vi "1553 Channels to Channel Handles.vi"(8 "error in":errorcluster, 10 "1553 channels":T5[](array[typedef]), 11 "Ballard MIL-STD 1553 custom device in":T2 format="%.0x") -> (0 "error out":errorcluster, 1 "Tx Channels":T2[](array[typedef]) format="%.0x", 2 "Rx Channels":T2[](array[typedef]) format="%.0x", 3 "Ballard MIL-STD 1553 custom device out":T2 format="%.0x", 4 "TX Messages":T1[](array[typedef]) {"Message Section Handle" format="%.0x"; "Parameter Channel Handles" format="%.0x"}, 6 "RX Messages":T1[](array[typedef]) {"Message Section Handle" format="%.0x"; "Parameter Channel Handles" format="%.0x"})   [LabVIEW 2020, in "AIM MIL-STD-1553 Engine.lvlib" / "Implementation.lvlib" / "Execution Unit.lvclass"]
uses:
  Execution Unit.lvclass
  <vilib>/NI VeriStand/Custom Device API/Custom Device Item Ref.ctl
  <vilib>/NI VeriStand/Custom Device API/Custom Device API.lvlib
  1553 Channel Handles.ctl
  Scripting/AIM MIL-STD-1553 Scripting.lvlib
  Parameter Handles.ctl
  Message Handles.ctl
  Shared/Error Count Channel Refs.ctl
  Shared/Direction.ctl
  Custom Device/Compiled Message.ctl
  Custom Device/Custom Device.lvlib
  Shared/Parameter Definition.ctl
  Shared/Address.ctl
  Shared/Terminal Endpoint.ctl
  Shared/Message Type.ctl
  Shared/Message Definition.ctl
  Shared/1553 Channel.ctl
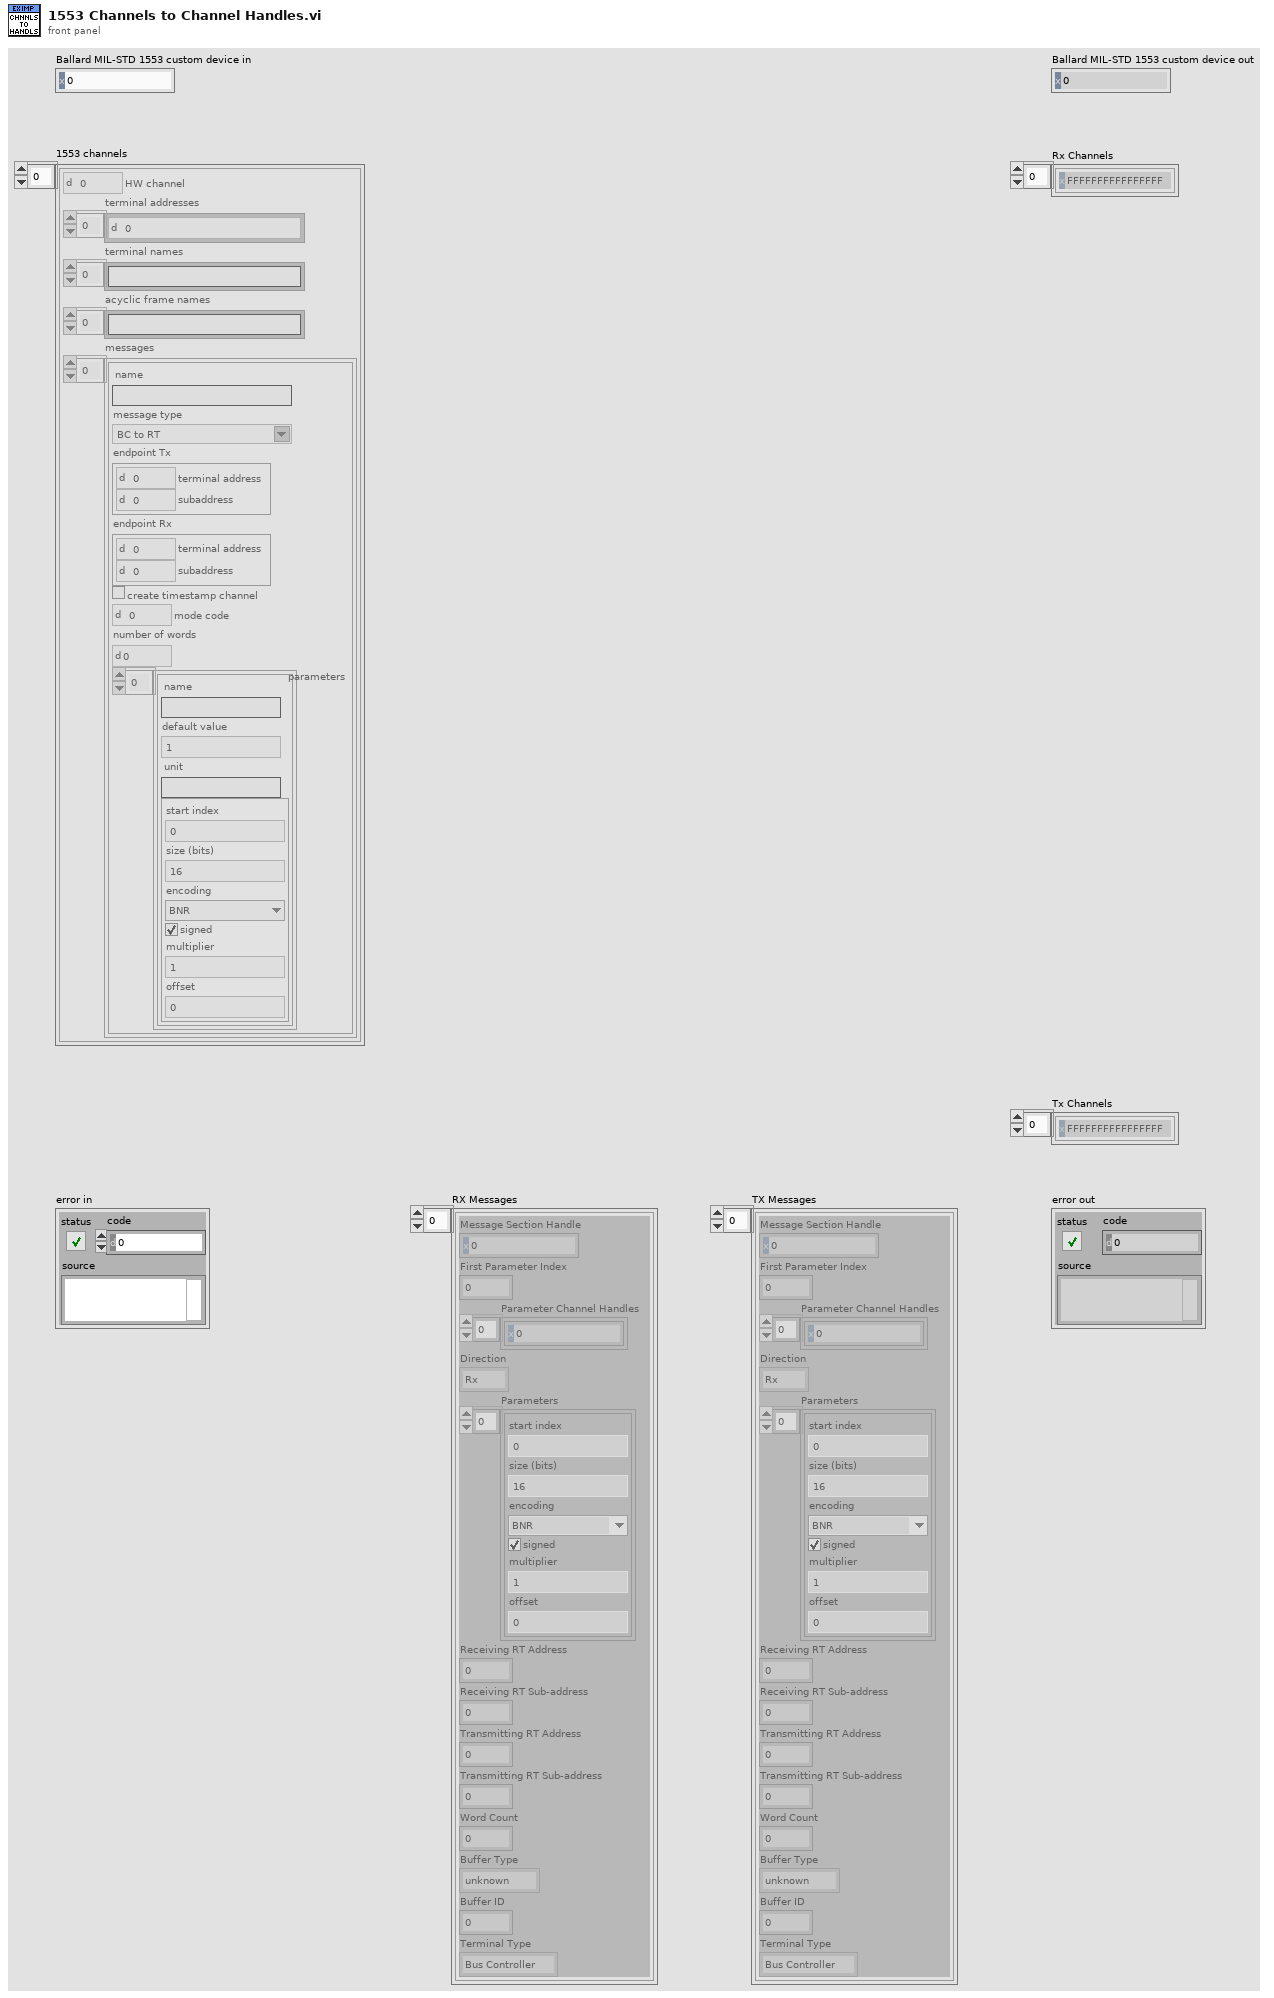
[diagram p1: front panel]
types:
  T1 = typedef "AIM MIL-STD-1553 Engine.lvlib/Custom Device.lvlib/Compiled Message.ctl" = cluster{"Message Section Handle":T2, "First Parameter Index":i32, "Parameter Channel Handles":T2[], "Direction":T3, "Parameters":T4[], "Receiving RT Address":u8, "Receiving RT Sub-address":u8, "Transmitting RT Address":u8, "Transmitting RT Sub-address":u8, "Word Count":u8, "Buffer Type":enum16{"unknown", "BC Message Buffer", "RT Message Buffer"}, "Buffer ID":u16, "Terminal Type":enum16{"Bus Controller", "Remote Terminal"}}
  T2 = typedef "Custom Device API.lvlib/Custom Device Item Ref.ctl" = u64
  T3 = typedef "Direction.ctl" = enum16{"Rx", "Tx"}
  T4 = typedef "Parameter Definition.ctl" = cluster{"start index":i32, "size (bits)":i32, "encoding":enum16{"BNR", "BCD", "Discrete"}, "signed":bool, "multiplier":dbl, "offset":dbl}
  T5 = typedef "1553 Channel.ctl" = cluster{"HW channel":u16, "terminal addresses":T6[], "terminal names":string[], "acyclic frame names":string[], "messages":T7[]}
  T6 = typedef "Address.ctl" = u16
  T7 = typedef "Message Definition.ctl" = cluster{"name":string, "message type":T8, "endpoint Tx":T9, "endpoint Rx":T9, "create timestamp channel":bool, "mode code":u16, "number of words":u16, "parameters":cluster{"name":string, "default value":dbl, "unit":string, "parameter definition":T4}[]}
  T8 = typedef "Message Type.ctl" = string
  T9 = typedef "Terminal Endpoint.ctl" = cluster{"terminal address":T6, "subaddress":T6}
  T10 = typedef "AIM MIL-STD-1553 Engine.lvlib/Implementation.lvlib/Execution Unit.lvclass/1553 Channel Handles.ctl" = cluster{"messages":T11[], "error count channel refs":T13, "terminal status channels":T2[]}
  T11 = typedef "AIM MIL-STD-1553 Engine.lvlib/Implementation.lvlib/Execution Unit.lvclass/Message Handles.ctl" = cluster{"parameters":T12[], "timestamps":T2[], "Tx status handles":T2[], "Rx status handles":T2[]}
  T12 = typedef "AIM MIL-STD-1553 Engine.lvlib/Implementation.lvlib/Execution Unit.lvclass/Parameter Handles.ctl" = cluster{"Tx channel handle":T2, "RxRT channel handle":T2, "RxBC channel handle":T2}
  T13 = typedef "Error Count Channel Refs.ctl" = cluster{"general protocol":T2, "improper number of words":T2, "Manchester":T2, "monitor":T2, "parity":T2, "unconfigured frames":T2, "word":T2, "wrong sync":T2}
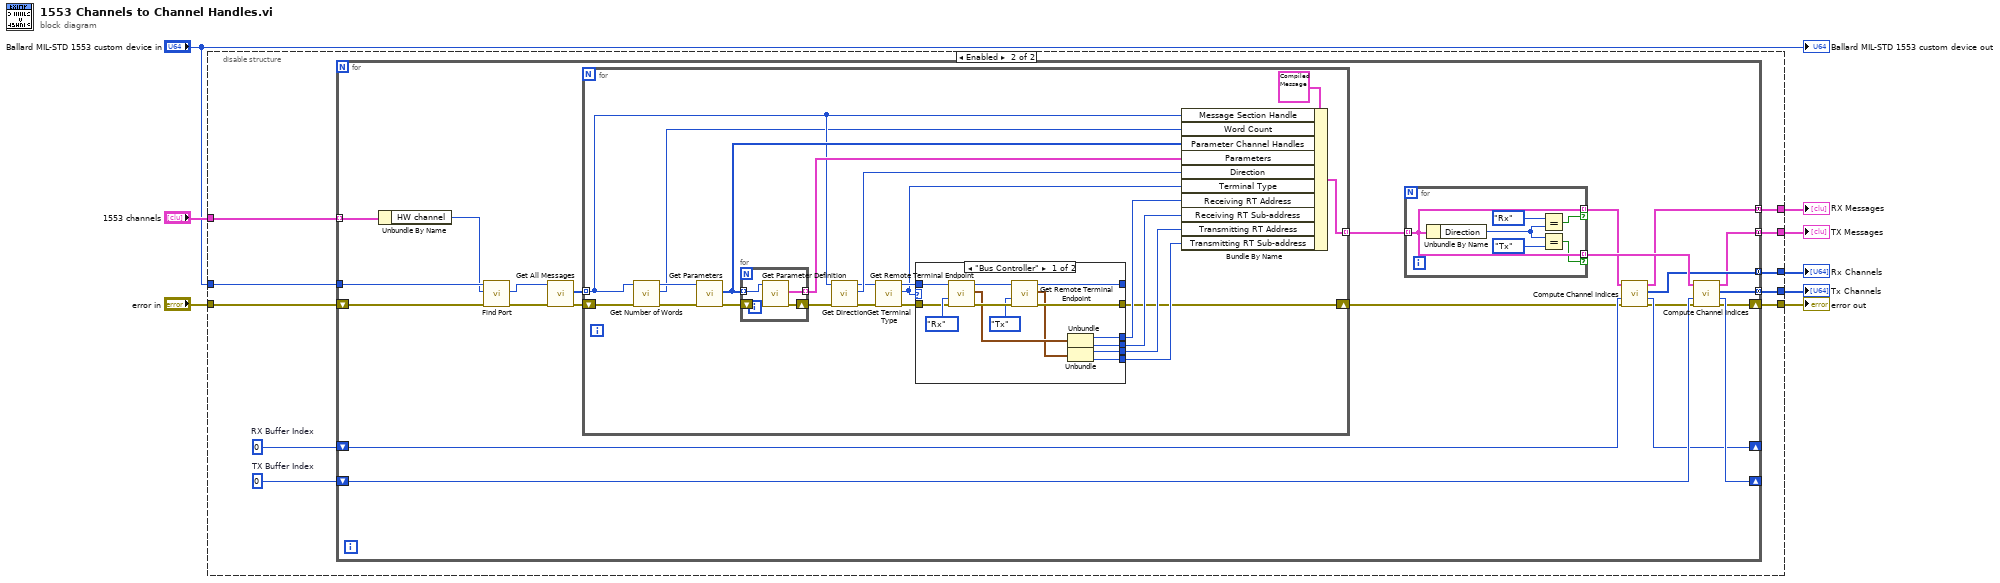
[diagram p0: block diagram]
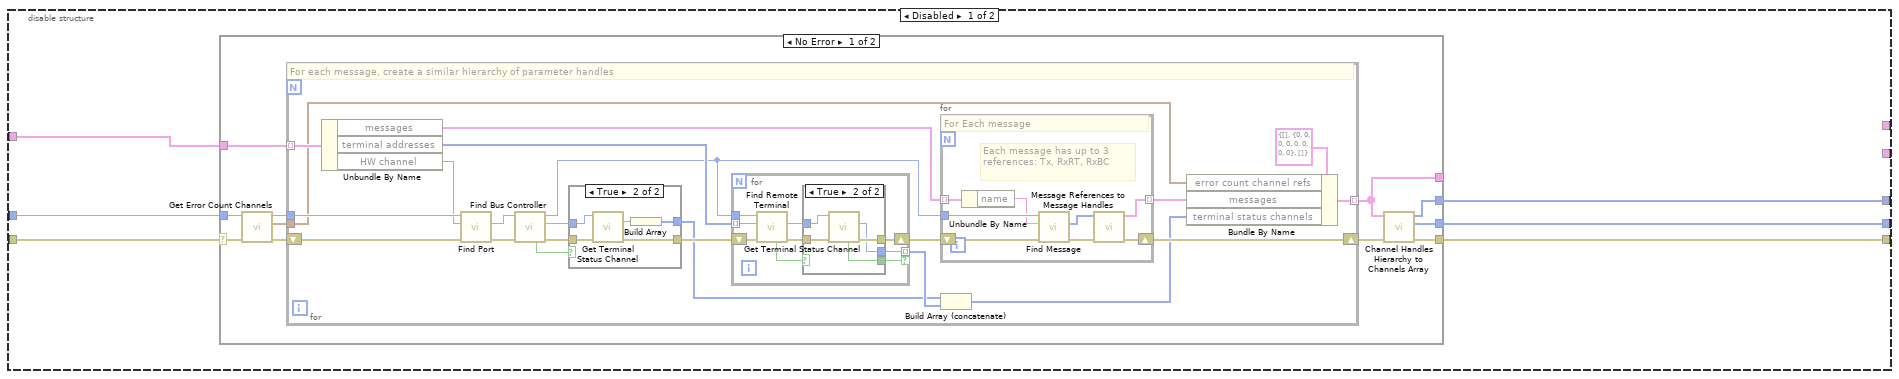
[diagram p2: hidden frame]
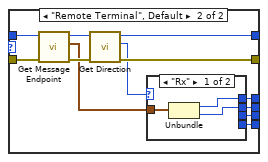
[diagram p6: hidden frame]
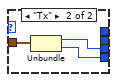
[diagram p7: hidden frame]
diagram:
  n1 = disable-structure shown="Enabled" {
    disable-tunnel: "error in" -> [w14 w89]
    disable-tunnel: "1553 channels" -> [w13 w87]
    disable-tunnel: [w12 w88] -> w6
    disable-tunnel: [w11 w85] -> w5
    disable-tunnel: [w10 w82] -> w4
    disable-tunnel: "Ballard MIL-STD 1553 custom device in" -> [w9 w86]
    disable-tunnel: [_ w81] -> w2
    disable-tunnel: [_ w80] -> w1
    frame Disabled {
      n2 = case shown="No Error" w14 {
        selector: w14 -> [w18 w79]
        tunnel: w13 -> [w25 _]
        tunnel: [w23 w79] -> w12
        tunnel: [w22 _] -> w11
        tunnel: [w21 _] -> w10
        tunnel: [w20 _] -> _
        tunnel: w9 -> [w17 _]
        frame No Error {
          n3 = call "Get Error Count Channels.vi"("error in"=w18, "Ballard MIL-STD-1553 custom device in"=w17) -> ("error out"=w19:errorcluster, "error count channel refs"=w15:T13, "Ballard MIL-STD-1553 custom device out"=w16:T2)  [unwired: 6 in, 1 out]
          n4 = for {
            tunnel: w25 -> [w42] mode=indexing
            shift-right: [w43] -> w24
            shift-left: w19 -> [w40]
            tunnel: [w44] -> w20 mode=indexing
            tunnel: w16 -> [w41]
            tunnel: w15 -> [w26]
            # "For each message, create a similar hierarchy of parameter handles"
            n5 = Unbundle By Name(w42) -> ("messages"=w47:T7[], "terminal addresses"=w38:T6[], "HW channel"=w27:u16)
            n6 = call "Find Port.vi"("error in"=w40, "port number"=w27, "Ballard MIL-STD 1553 custom device in"=w41) -> ("error out"=w36:errorcluster, "port"=w35:T2)  [unwired: 5 in, 2 out]
            n7 = call "Find Bus Controller.vi"("error in"=w36, "port in"=w35) -> ("error out"=w30:errorcluster, "bus controller"=w32:T2, "port out"=w33:T2, "found?"=w31:bool)  [unwired: 6 in]
            n8 = case shown="True" w31 {
              tunnel: w32 -> [_ w53]
              tunnel: w30 -> [w48 w51]
              tunnel: [w48 w50] -> w29
              tunnel: [_ w49] -> w28
              frame False {
              }
              frame True {
                n9 = call "Get Terminal Status Channel.vi"("error in"=w51, "terminal in"=w53) -> ("error out"=w50:errorcluster, "status channel"=w52:T2)  [unwired: 6 in, 2 out]
                n10 = Build Array(w52) -> (w49:T2[])
              }
            }
            n11 = for {
              shift-right: [w59] -> w39
              shift-left: w29 -> [w61]
              tunnel: w33 -> [w62]
              tunnel: w38 -> [w60] mode=indexing
              tunnel: [w55] -> w37 mode=indexing if=w54
              n12 = call "Find Remote Terminal.vi"("error in"=w61, "terminal address"=w60, "port in"=w62) -> ("error out"=w56:errorcluster, "remote terminal"=w57:T2, "found?"=w58:bool)  [unwired: 5 in, 1 out]
              n13 = case shown="True" w58 {
                selector: w58 -> [w63 _]
                tunnel: w57 -> [w64 w70]
                tunnel: w56 -> [w65 w69]
                tunnel: [w65 w68] -> w59
                tunnel: [w64 w67] -> w55
                tunnel: [w63 w66] -> w54
                frame False {
                }
                frame True {
                  n14 = call "Get Terminal Status Channel.vi"("error in"=w69, "terminal in"=w70) -> ("error out"=w68:errorcluster, "status channel"=w67:T2, "found?"=w66:bool)  [unwired: 6 in, 1 out]
                }
              }
            }
            n15 = for {
              tunnel: w47 -> [w77] mode=indexing
              shift-right: [w72] -> w43
              shift-left: w39 -> [w78]
              tunnel: w33 -> [w76]
              tunnel: [w71] -> w45 mode=indexing
              # "Each message has up to 3 references: Tx, RxRT, RxBC"
              # "For Each message"
              n16 = Unbundle By Name(w77) -> ("name"=w75:string)
              n17 = call "Find Message.vi"("error in"=w78, "message name"=w75, "port in"=w76) -> ("error out"=w74:errorcluster, "message refs"=w73:T2[])  [unwired: 5 in, 2 out]
              n18 = call "Message References to Message Handles.vi"("error in"=w74, "message refs"=w73) -> ("error out"=w72:errorcluster, "message handles"=w71:T11)  [unwired: 8 in]
            }
            n19 = Build Array (concatenate)(w28, w37) -> (w34:T2[])
            n20 = Bundle By Name(cluster=T10 {"messages"=[], "error count channel refs"={"general protocol"=0, "improper number of words"=0, "Manchester"=0, "monitor"=0, "parity"=0, "unconfigured frames"=0, "word"=0, "wrong sync"=0}, "terminal status channels"=[]} ("1553 channel handles"), "error count channel refs"=w26, "messages"=w45, "terminal status channels"=w34) -> (w44:T10)
          }
          n21 = call "Channel Handles Hierarchy to Channels Array.vi"("error in"=w24, "1553 channel handles"=w20) -> ("error out"=w23:errorcluster, "Tx Channels"=w22:T2[], "Rx Channels"=w21:T2[])  [unwired: 7 in]
        }
        frame Error {
        }
      }
    }
    frame Enabled {
      w83 = 0  # RX Buffer Index
      w84 = 0  # TX Buffer Index
      n22 = for {
        shift-right: [w92] -> w88
        shift-left: w89 -> [w110]
        tunnel: w87 -> [w111] mode=indexing
        tunnel: w86 -> [w109]
        tunnel: [w100] -> w85 mode=concatenating
        shift-right: [w96] -> _
        shift-left: w83 -> [w97]
        shift-right: [w98] -> _
        shift-left: w84 -> [w99]
        tunnel: [w95] -> w82 mode=concatenating
        tunnel: [w91] -> w81 mode=concatenating
        tunnel: [w90] -> w80 mode=concatenating
        n23 = Unbundle By Name(w111) -> ("HW channel"=w108:u16)
        n24 = call "Find Port.vi"("error in"=w110, "port number"=w108, "Ballard MIL-STD 1553 custom device in"=w109) -> ("error out"=w107:errorcluster, "port"=w106:T2)  [unwired: 5 in, 2 out]
        n25 = call "Get All Messages.vi"("error in"=w107, "port in"=w106) -> ("error out"=w105:errorcluster, "messages"=w104:T2[])  [unwired: 7 in, 1 out]
        n26 = for {
          shift-right: [w124] -> w94
          shift-left: w105 -> [w122]
          tunnel: w104 -> [w123] mode=indexing
          tunnel: [w139] -> w103 mode=indexing
          n27 = call "Get Number of Words.vi"("error in"=w122, "message in"=w123) -> ("error out"=w121:errorcluster, "number of words"=w119:u16, "message out"=w120:T2)  [unwired: 7 in]
          n28 = call "Get Parameters.vi"("error in"=w121, "message in"=w120) -> ("error out"=w136:errorcluster, "parameters"=w135:T2[])  [unwired: 7 in, 1 out]
          n29 = for {
            shift-right: [w175] -> w133
            shift-left: w136 -> [w174]
            tunnel: w135 -> [w173] mode=indexing
            tunnel: [w172] -> w134 mode=indexing
            n30 = call "Get Parameter Definition.vi"("error in"=w174, "parameter in"=w173) -> ("error out"=w175:errorcluster, "parameter definition"=w172:T4)  [unwired: 7 in, 1 out]
          }
          n31 = call "Get Direction.vi"("error in"=w133, "message in"=w123) -> ("error out"=w130:errorcluster, "direction"=w137:T3, "message out"=w129:T2)  [unwired: 6 in, 1 out]
          n32 = call "Get Terminal Type.vi"("error in"=w130, "message in"=w129) -> ("error out"=w132:errorcluster, "terminal type"=w118:enum16{"Bus Controller", "Remote Terminal"}, "message out"=w131:T2)  [unwired: 7 in]
          n33 = case shown="\"Bus Controller\"" w118 {
            tunnel: [w147 w163] -> _
            tunnel: [w146 w162] -> w124
            tunnel: w131 -> [w153 w159]
            tunnel: w132 -> [w151 w158]
            tunnel: [w140 w157] -> w125
            tunnel: [w141 w156] -> w126
            tunnel: [w144 w155] -> w127
            tunnel: [w145 w154] -> w128
            frame "Bus Controller" {
              n34 = call "Get Remote Terminal Endpoint.vi"("error in"=w151, "direction"=Direction."Rx", "message in"=w153) -> ("error out"=w150:errorcluster, "remote terminal"=w143:T9, "message out"=w148:T2)  [unwired: 5 in, 1 out]
              n35 = call "Get Remote Terminal Endpoint.vi"("error in"=w150, "direction"=Direction."Tx", "message in"=w148) -> ("error out"=w146:errorcluster, "remote terminal"=w142:T9, "message out"=w147:T2)  [unwired: 5 in, 1 out]
              n36 = Unbundle(w143) -> ("terminal address"=w145:T6, "subaddress"=w144:T6)
              n37 = Unbundle(w142) -> ("terminal address"=w141:T6, "subaddress"=w140:T6)
            }
            frame "Remote Terminal", Default {
              n38 = call "Get Message Endpoint.vi"("error in"=w158, "message in"=w159) -> ("error out"=w164:errorcluster, "message endpoint"=w160:T9, "message out"=w165:T2)  [unwired: 7 in]
              n39 = call "Get Direction.vi"("error in"=w164, "message in"=w165) -> ("error out"=w162:errorcluster, "direction"=w161:T3, "message out"=w163:T2)  [unwired: 6 in, 1 out]
              n40 = case shown="\"Rx\"" w161 {
                tunnel: w160 -> [w168 w171]
                tunnel: [w167 _] -> w154
                tunnel: [w166 _] -> w155
                tunnel: [_ w170] -> w156
                tunnel: [_ w169] -> w157
                frame "Rx" {
                  n41 = Unbundle(w168) -> ("terminal address"=w167:T6, "subaddress"=w166:T6)
                }
                frame "Tx" {
                  n42 = Unbundle(w171) -> ("terminal address"=w170:T6, "subaddress"=w169:T6)
                }
              }
            }
          }
          n43 = Bundle By Name(cluster=T1 {"Message Section Handle"=18446744073709551615, "First Parameter Index"=0, "Parameter Channel Handles"=[], "Direction"=enum."Rx", "Parameters"=[], "Receiving RT Address"=0, "Receiving RT Sub-address"=0, "Transmitting RT Address"=0, "Transmitting RT Sub-address"=0, "Word Count"=0, "Buffer Type"=enum."unknown", "Buffer ID"=0, "Terminal Type"=enum."Bus Controller"}, "Message Section Handle"=w123, "Word Count"=w119, "Parameter Channel Handles"=w135, "Parameters"=w134, "Direction"=w137, "Terminal Type"=w118, "Receiving RT Address"=w128, "Receiving RT Sub-address"=w127, "Transmitting RT Address"=w126, "Transmitting RT Sub-address"=w125) -> (w139:T1)
        }
        n44 = for {
          tunnel: w103 -> [w117] mode=indexing
          tunnel: [w117] -> w101 mode=indexing if=w113
          tunnel: [w117] -> w102 mode=indexing if=w112
          n45 = Unbundle By Name(w117) -> ("Direction"=w116:T3)
          n46 = Equal?(x=Direction."Rx", y=w116) -> (x = y?=w113:bool)
          n47 = Equal?(x=w116, y=Direction."Tx" ("x")) -> (x = y?=w112:bool)
        }
        n48 = call "Compute Channel Indices.vi"("error in (no error)"=w94, "Next Index in"=w97, "Messages in"=w101) -> ("error out"=w93:errorcluster, "Next Index out"=w96:i32, "Channel Handles"=w95:T2[], "Messages out"=w91:T1[])  [unwired: 5 in]
        n49 = call "Compute Channel Indices.vi"("error in (no error)"=w93, "Next Index in"=w99, "Messages in"=w102) -> ("error out"=w92:errorcluster, "Next Index out"=w98:i32, "Channel Handles"=w100:T2[], "Messages out"=w90:T1[])  [unwired: 5 in]
      }
    }
  }
  "Rx Channels" <- w4
  "error out" <- w6
  "Tx Channels" <- w5
  "RX Messages" <- w2
  "TX Messages" <- w1
  "Ballard MIL-STD 1553 custom device out" <- "Ballard MIL-STD 1553 custom device in"
